vi "WriteAppLog.vi"() -> ()   [LabVIEW 2024]
panel:
  out "error out":errorcluster
  in  "error in":errorcluster
  in  "String To Write":string
  out "Is Valid?":bool
  out "AppLog Path":path
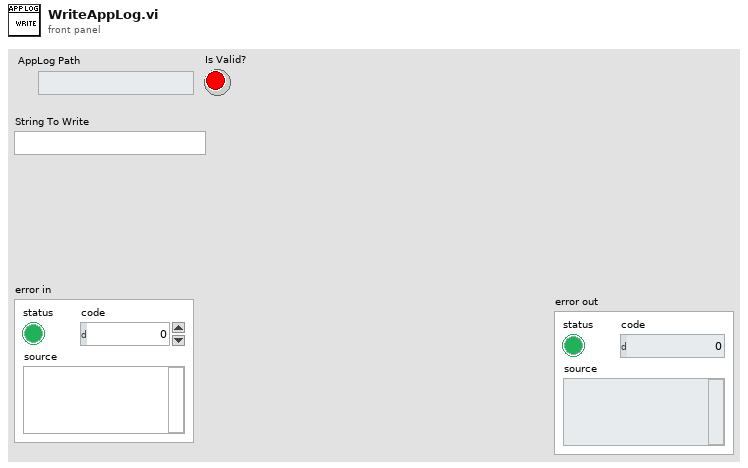
[diagram p1: front panel]
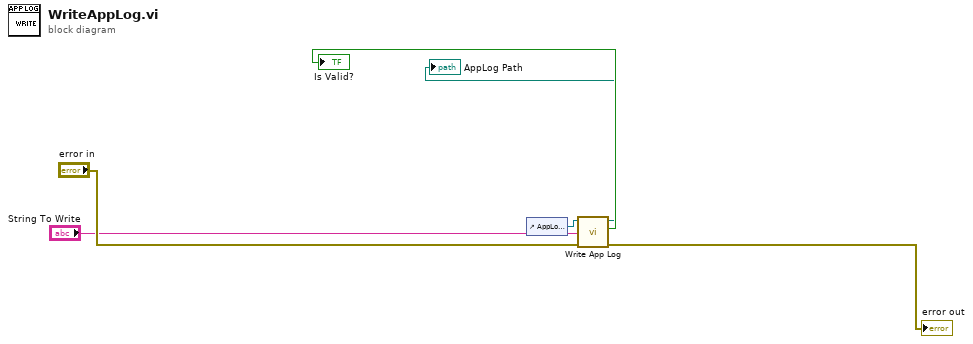
[diagram p0: block diagram]
diagram:
  n1 = control-ref of="AppLog Path"() -> (w3:refnum<vi>)
  n2 = call "Write App Log.vi"("error in (no error)"="error in", "String To Write"="String To Write", "Path in"=w3) -> ("error out"=→"error out":errorcluster, "Is Valid?"=→"Is Valid?":bool, "AppLog Path"=→"AppLog Path":path)  [unwired: 6 in]
